vi "SVPO Limit Testing (Scalar) (DBL) with IC.vi"(7 "reset? (F)":bool, 8 "initial conditions":T1, 9 "lower limit":dbl=-inf format="%.2f", 10 "upper limit":dbl=inf format="%.2f", 11 "value in":dbl=inf format="%.2f") -> (0 "final conditions":T1, 1 "lower limit clearance":dbl format="%.6f", 2 "upper limit clearance":dbl format="%.6f", 3 "test passed?":bool)   [LabVIEW 2017, in "SoundVib_LimitTest.lvlib"]
doc: "Performs limit testing on single-precision waveforms, single-precision scaled arrays, or double-precision scalar measurements. You can specify an upper and lower boundary of the envelope to define a pass range. This VI uses the defined pass range to test the input signal. VI outputs apply to all the tests since the last VI reset. Use this VI on embedded targets that have limited computational resources. Wire data to the <B>value in</B> input to determine the polymorphic instance to use or manually select the instance."
uses:
  <vilib>/addons/Sound and Vibration/svt_Limit Test/SoundVib_LimitTest.lvlib
  <vilib>/addons/_NISVFA/_Shared subVIs/Controls/svc_DBL Limit State.ctl
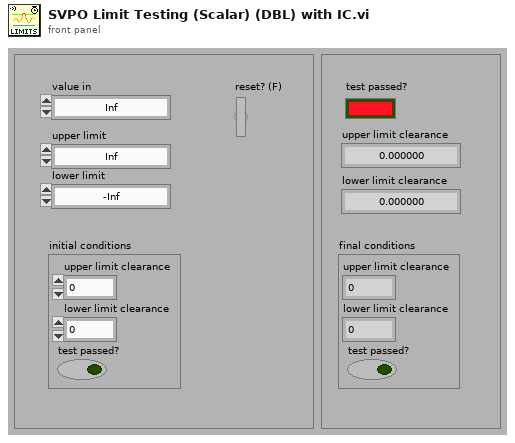
[diagram p1: front panel]
types:
  T1 = typedef "svc_DBL Limit State.ctl" = cluster{"upper limit clearance":dbl, "lower limit clearance":dbl, "test passed?":bool}
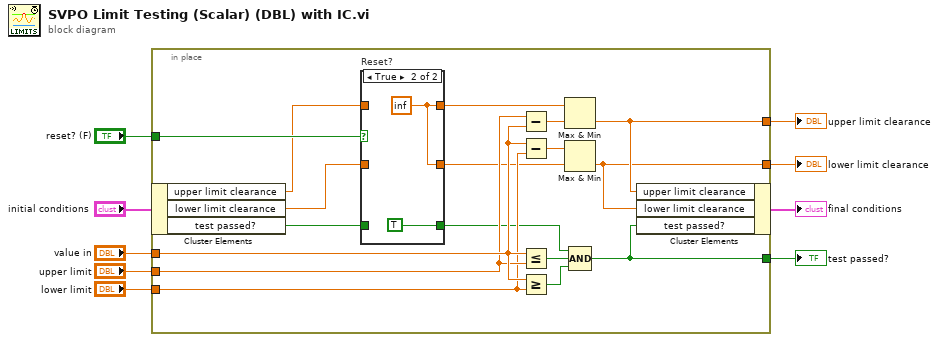
[diagram p0: block diagram]
diagram:
  n1 = in-place {
    in-place-border: "value in" -> [w26]
    in-place-border: "upper limit" -> [w25]
    in-place-border: "lower limit" -> [w24]
    in-place-border: [w12] -> w6
    in-place-border: [w11] -> w5
    in-place-border: [w10] -> w4
    in-place-border: "reset? (F)" -> [w23]
    n2 = in-place-cluster #1("initial conditions") -> ("upper limit clearance"=w15:dbl, "lower limit clearance"=w14:dbl, "test passed?"=w13:bool)
    n3 = case "Reset?" shown="True" w23 {
      tunnel: w15 -> [w29 _]
      tunnel: [w29 w30] -> w22
      tunnel: w14 -> [w28 _]
      tunnel: [w28 w30] -> w21
      tunnel: w13 -> [w27 _]
      tunnel: [w27 TRUE] -> w16
      frame False {
      }
      frame True {
        w30 = inf
      }
    }
    n4 = Subtract(x=w25, y=w26) -> (x-y=w18:dbl)
    n5 = Subtract(x=w26, y=w24) -> (x-y=w17:dbl)
    n6 = Less Or Equal?(x=w26, y=w25) -> (x <= y?=w20:bool)
    n7 = Greater Or Equal?(x=w26, y=w24) -> (x >= y?=w19:bool)
    n8 = Max & Min(x=w22, y=w18) -> (min(x,y)=w12:dbl)  [unwired: 1 out]
    n9 = Max & Min(x=w17, y=w21) -> (min(x,y)=w11:dbl)  [unwired: 1 out]
    n10 = Compound Arithmetic op=AND(w16, w20, w19) -> (w10:bool)
    n11 = in-place-cluster #1("upper limit clearance"=w12, "lower limit clearance"=w11, "test passed?"=w10) -> (→"final conditions":T1)
  }
  "test passed?" <- w4
  "upper limit clearance" <- w6
  "lower limit clearance" <- w5
